vi "AddConnectionWindow.vi"(8 "error in (no error)":errorcluster, 11 "TCP_Server in":refnum<class "TCP_Server.lvclass">) -> (0 "error out":errorcluster, 3 "TCP_Server out":refnum<class "TCP_Server.lvclass">)   [LabVIEW 2023, in "TCP_Server.lvlib" / "TCP_Server.lvclass"]
uses:
  TCP_Server.lvclass
  C:/Program Files (x86)/National Instruments/LabVIEW 2023/vi.lib/ActorFramework/Actor/Actor.lvclass
  TCP_Client_Window/TCP_Client_Window/TCP_Client_Window.lvclass
  TCP_Server.lvclass/TCP_Server.ctl
  TCP_Client_Window/TCP_Client_Window Messages/UpdateWindowTitle Msg/UpdateWindowTitle Msg.lvclass/UpdateWindowTitle Msg.ctl
  <vilib>/ActorFramework/Message Enqueuer/Message Enqueuer.lvclass/Message Enqueuer.ctl
  TCP_Client_Window/TCP_Client_Window Messages/Write Connection Number Msg/Write Connection Number Msg.lvclass/Write Connection Number Msg.ctl
  <vilib>/ActorFramework/Message Enqueuer/Enqueue.vi
  TCP_Client_Window/TCP_Client_Window Messages/UpdateWindowTitle Msg/UpdateWindowTitle Msg.lvclass
  C:/Program Files (x86)/National Instruments/LabVIEW 2023/vi.lib/ActorFramework/Message/Message.lvclass
  TCP_Client_Window/TCP_Client_Window Messages/Write Connection Number Msg/Write Connection Number Msg.lvclass
  <vilib>/ActorFramework/Message Priority Queue/Priority Enqueue.vi
  <vilib>/ActorFramework/Actor/Actor.lvclass
  TCP_Client_Window/TCP_Client_Window Messages/Write Error Logger's Enqueuer Msg/Write Error Logger's Enqueuer Msg.lvclass
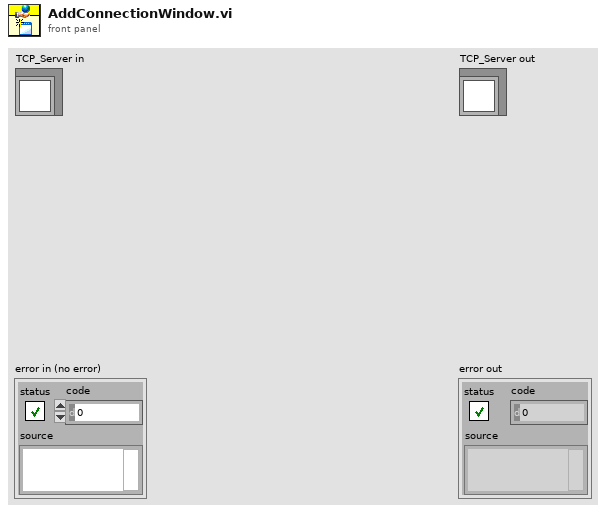
[diagram p1: front panel]
types:
  T1 = typedef "TCP_Server.lvlib/ServerConnection.ctl" = cluster{"Connection Handlers's Enqueuer":refnum<class "Message Enqueuer.lvclass">, "Connection Window's Enqueuer":refnum<class "Message Enqueuer.lvclass">, "Connection Information":T2}
  T2 = typedef "TCP_Listener.lvlib/ConnectionInformation.ctl" = cluster{"Connection number":i32, "Remote Address":string, "Remote Port":u16, "Connection ID":refnum<k5>}
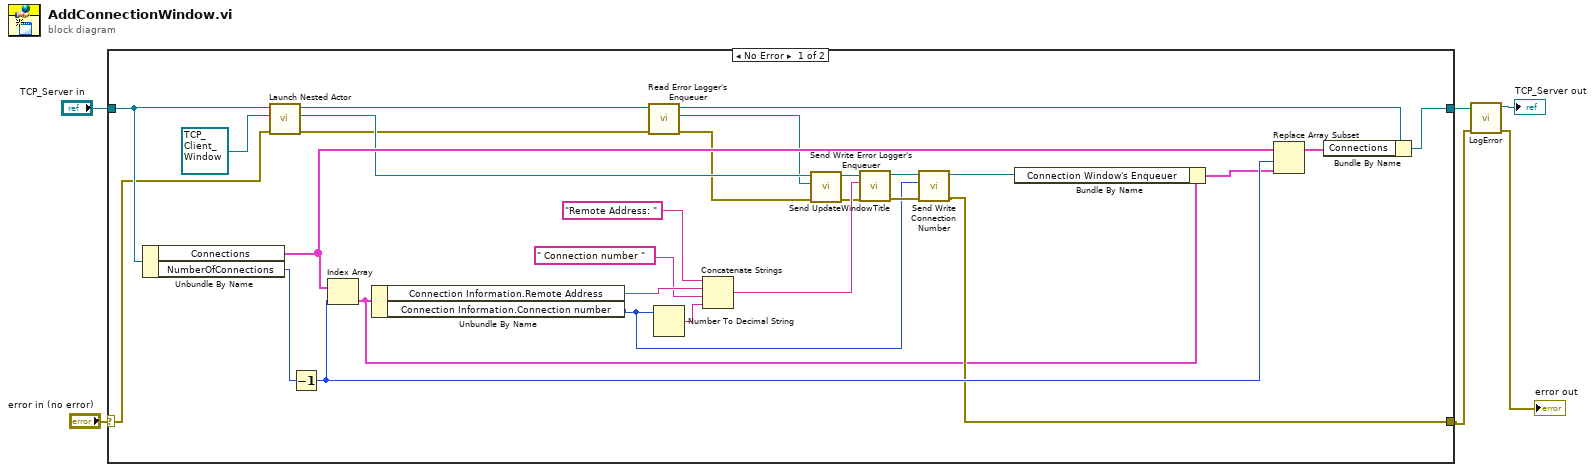
[diagram p0: block diagram]
diagram:
  n1 = case shown="No Error" "error in (no error)" {
    selector: "error in (no error)" -> [w9 w36]
    tunnel: [w18 w36] -> w2
    tunnel: [w24 w35] -> w4
    tunnel: "TCP_Server in" -> [w33 w35]
    frame No Error {
      n2 = Unbundle By Name(w33) -> ("Connections"=w23:T1[], "NumberOfConnections"=w32:i32)
      n3 = call <vilib>:"Launch Nested Actor.vi"("error in (no error)"=w9, "Nested Actor"=refnum<class "TCP_Client_Window.lvclass"> refnum ("TCP_Client_Window.lvlib:TCP_Client_Window.lvclass"), "Caller Actor in"=w33) -> ("error out"=w8:errorcluster, "Nested Actor's Enqueuer"=w15:refnum<class "Message Enqueuer.lvclass">, "Caller Actor out"=w12:refnum<class "TCP_Server.lvclass">)  [unwired: 6 in]
      n4 = Decrement(x=w32) -> (x-1=w26:i32)
      n5 = Index Array(array=w23, index=w26) -> (element=w17:T1)
      n6 = Unbundle By Name(w17) -> ("Connection Information.Remote Address"=w30:string, "Connection Information.Connection number"=w16:i32)
      n7 = call "Read Error Logger's Enqueuer.vi"("error in (no error)"=w8, "TCP_Server in"=w12) -> ("error out"=w7:errorcluster, "Actor Framework:Message Enqueuer"=w10:refnum<class "Message Enqueuer.lvclass">, "TCP_Server out"=w11:refnum<class "TCP_Server.lvclass">)  [unwired: 7 in]
      n8 = Number To Decimal String(number=w16) -> (decimal integer string=w28:string)  [unwired: 1 in]
      n9 = Concatenate Strings("Remote Address: " ("string"), w30, " Connection number " ("string"), w28) -> (w27:string)
      n10 = call "Send Write Error Logger's Enqueuer.vi"("error in (no error)"=w7, "Actor Framework:Message Enqueuer"=w10, "Message Enqueuer"=w15) -> ("error out"=w13:errorcluster, "Message Enqueuer out"=w14:refnum<class "Message Enqueuer.lvclass">)  [unwired: 7 in]
      n11 = call "Send UpdateWindowTitle.vi"("error in (no error)"=w13, "WindowTitle"=w27, "Message Enqueuer"=w14) -> ("error out"=w19:errorcluster, "Message Enqueuer out"=w21:refnum<class "Message Enqueuer.lvclass">)  [unwired: 7 in]
      n12 = call "Send Write Connection Number.vi"("error in (no error)"=w19, "Connection Number"=w16, "Message Enqueuer"=w21) -> ("error out"=w18:errorcluster, "Message Enqueuer out"=w20:refnum<class "Message Enqueuer.lvclass">)  [unwired: 7 in]
      n13 = Bundle By Name(cluster=w17, "Connection Window's Enqueuer"=w20) -> (w22:T1)
      n14 = Replace Array Subset(array=w23, new element=w22, index=w26) -> (w25:T1[])
      n15 = Bundle By Name(cluster=w11, "Connections"=w25) -> (w24:refnum<class "TCP_Server.lvclass">)
    }
    frame Error {
    }
  }
  n16 = call "LogError.vi"("error in (no error)"=w2, "TCP_Server in"=w4) -> ("error out"=→"error out":errorcluster, "TCP_Server out"=→"TCP_Server out":refnum<class "TCP_Server.lvclass">)  [unwired: 8 in]
